vi "CalcStereoDist.vi"(2 "Image Height":i32, 3 "Image Width":i32, 4 "BlobData":T2(array[cluster])) -> (0 "Dist":cluster{"Distance":dbl, "Area":dbl}[](array[cluster]), 1 "Distance":T1(array[cluster]))   [LabVIEW 2011]
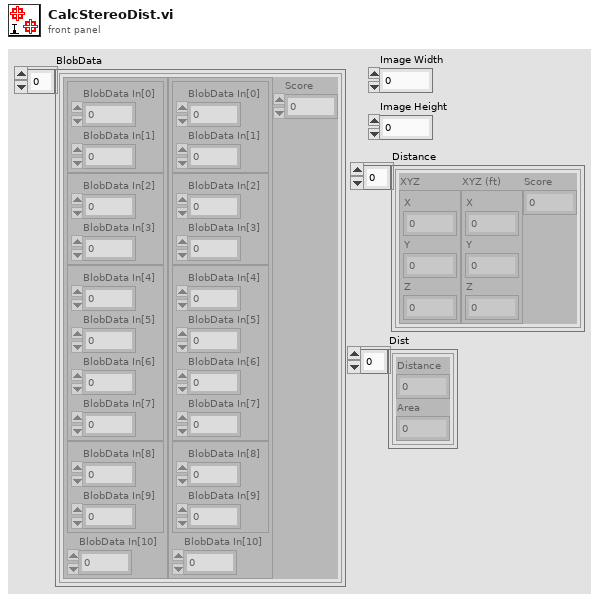
[diagram p1: front panel]
types:
  T1 = cluster{"XYZ":cluster{"X":dbl, "Y":dbl, "Z":dbl}, "XYZ (ft)":cluster{"X":dbl, "Y":dbl, "Z":dbl}, "Score":dbl}[]
  T2 = cluster{cluster{cluster{"BlobData In[0]":dbl, "BlobData In[1]":dbl}, cluster{"BlobData In[2]":dbl, "BlobData In[3]":dbl}, cluster{"BlobData In[4]":dbl, "BlobData In[5]":dbl, "BlobData In[6]":dbl, "BlobData In[7]":dbl}, cluster{"BlobData In[8]":dbl, "BlobData In[9]":dbl}, "BlobData In[10]":dbl}, cluster{cluster{"BlobData In[0]":dbl, "BlobData In[1]":dbl}, cluster{"BlobData In[2]":dbl, "BlobData In[3]":dbl}, cluster{"BlobData In[4]":dbl, "BlobData In[5]":dbl, "BlobData In[6]":dbl, "BlobData In[7]":dbl}, cluster{"BlobData In[8]":dbl, "BlobData In[9]":dbl}, "BlobData In[10]":dbl}, "Score":dbl}[]
  T3 = cluster{cluster{"BlobData In[0]":dbl, "BlobData In[1]":dbl}, cluster{"BlobData In[2]":dbl, "BlobData In[3]":dbl}, cluster{"BlobData In[4]":dbl, "BlobData In[5]":dbl, "BlobData In[6]":dbl, "BlobData In[7]":dbl}, cluster{"BlobData In[8]":dbl, "BlobData In[9]":dbl}, "BlobData In[10]":dbl}
  T4 = cluster{"BlobData In[0]":dbl, "BlobData In[1]":dbl}
  T5 = cluster{"XYZ":cluster{"X":dbl, "Y":dbl, "Z":dbl}, "XYZ (ft)":cluster{"X":dbl, "Y":dbl, "Z":dbl}, "Score":dbl}
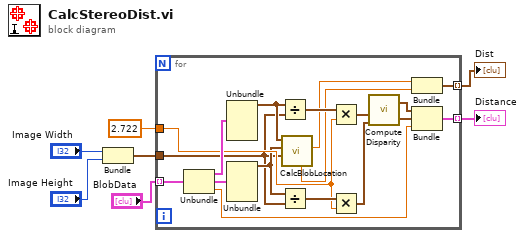
[diagram p0: block diagram]
diagram:
  n1 = Bundle("Image Width"="Image Width", "Image Height"="Image Height") -> (w4:cluster{"Image Width":i32, "Image Height":i32})  [unwired: 1 in]
  n2 = for {
    tunnel: "BlobData" -> [w22] mode=indexing
    tunnel: w4 -> [w11]
    tunnel: [w23] -> w3 mode=indexing
    tunnel: 2.722 -> [w14]
    tunnel: [w8] -> w1 mode=indexing
    n3 = Unbundle(w22) -> (w25:T3, w24:T3, "Score"=w21:dbl)
    n4 = Unbundle(w25) -> (w13:T4)  [unwired: 4 out]
    n5 = Unbundle(w24) -> (w12:T4)  [unwired: 4 out]
    n6 = Divide(x=w13, y=w11) -> (x/y=w20:cluster{dbl, dbl})
    n7 = Divide(x=w12, y=w11) -> (x/y=w19:cluster{dbl, dbl})
    n8 = call "CalcBlobLocation.vi"("ImageSize  (px)"=w11, "TargetBlob (px)"=w12, "RefBlob (px)"=w13) -> ("Distance"=w10:dbl, "Area"=w9:dbl)  [unwired: 4 in, 3 out]
    n9 = Multiply(x=w20, y=w14) -> (x*y=w16:cluster{dbl, dbl})
    n10 = Multiply(x=w19, y=w14) -> (x*y=w15:cluster{dbl, dbl})
    n11 = call "Compute Disparity.vi"("t"=w15, "r"=w16) -> ("XYZ (ft)"=w17:cluster{"X":dbl, "Y":dbl, "Z":dbl}, "XYZ"=w18:cluster{"X":dbl, "Y":dbl, "Z":dbl})  [unwired: 2 in]
    n12 = Bundle("Distance"=w10, "Area"=w9) -> (w8:cluster{"Distance":dbl, "Area":dbl})  [unwired: 1 in]
    n13 = Bundle("XYZ"=w18, "XYZ (ft)"=w17, "Score"=w21) -> (w23:T5)  [unwired: 1 in]
  }
  "Distance" <- w3
  "Dist" <- w1
